vi "Set Channel Enable Mask.vi"(8 "error in (no error)":errorcluster, 10 "Channel Enable":bool[](array[boolean])=[FALSE, FALSE, FALSE, FALSE, FALSE, FALSE, FALSE, FALSE, FALSE, FALSE, FALSE, FALSE, FALSE, FALSE, FALSE, FALSE, FALSE, FALSE], 11 "LINX-SN3218 in":refnum<class "LINX-SN3218.lvclass">) -> (0 "error out":errorcluster, 3 "LINX-SN3218 out":refnum<class "LINX-SN3218.lvclass">)   [LabVIEW 2020, in "LINX-SN3218.lvclass"]
uses:
  LINX-SN3218.lvclass
  LINX I2C/LINX I2C.lvclass
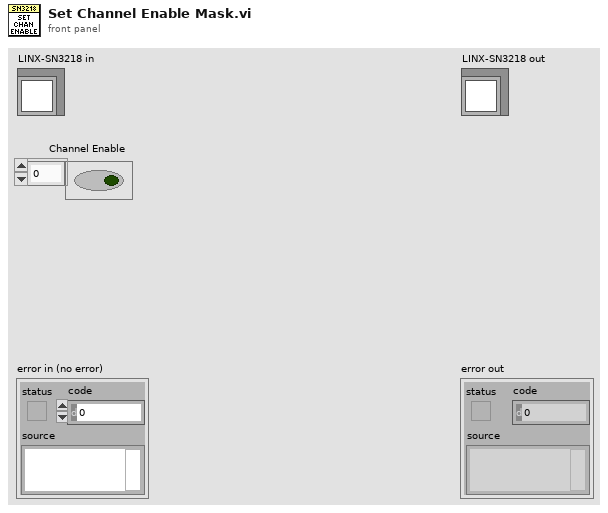
[diagram p1: front panel]
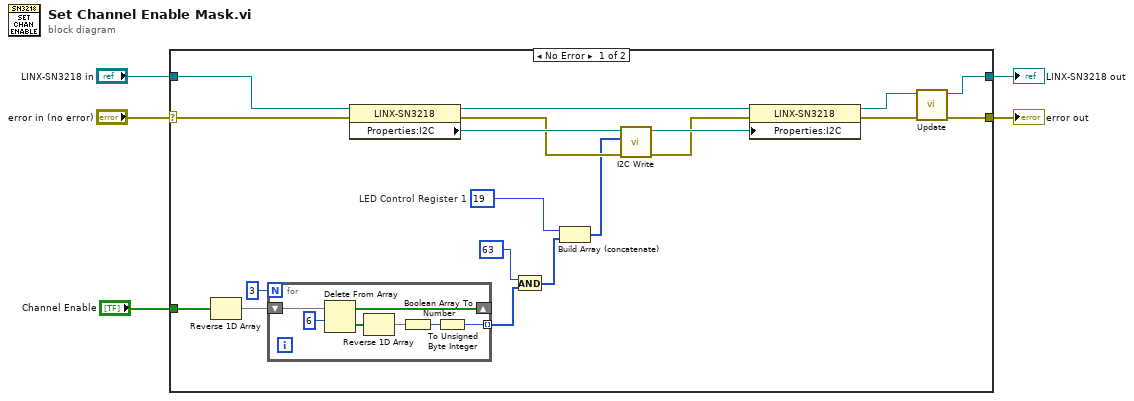
[diagram p0: block diagram]
diagram:
  n1 = case shown="No Error" "error in (no error)" {
    selector: "error in (no error)" -> [w22 w33]
    tunnel: [w11 w33] -> w4
    tunnel: [w10 w32] -> w2
    tunnel: "LINX-SN3218 in" -> [w24 w32]
    tunnel: "Channel Enable" -> [w9 _]
    frame No Error {
      w17 = u8 19  # LED Control Register 1
      n2 = Reverse 1D Array(array=w9) -> (reversed array=w6:bool[])
      n3 = for {
        N: 3 -> [_]
        shift-right: [w30] -> _
        shift-left: w6 -> [w31]
        tunnel: [w26] -> w7 mode=indexing
        n4 = Delete From Array(array=w31, length=6) -> (deleted portion=w28:bool[], array with subset deleted=w30:bool[])  [unwired: 1 in]
        n5 = Reverse 1D Array(array=w28) -> (reversed array=w25:bool[])
        n6 = Boolean Array To Number(Boolean array=w25) -> (number=w27:u32)
        n7 = To Unsigned Byte Integer(number=w27) -> (unsigned 8bit integer=w26:u8)
      }
      n8 = property class="LINX-SN3218"(reference=w24, error in=w22) -> (reference out=w21:refnum<class "LINX-SN3218.lvclass">, error out=w19:errorcluster, "Properties:I2C"=w23:refnum<class "LINX I2C.lvclass">)
      n9 = And(x=u8 63, y=w7) -> (x .and. y?=w14:u8[])
      n10 = Build Array (concatenate)(w17, w14) -> (w16:u8[])
      n11 = call "I2C Write.vi"("error in (no error)"=w19, "Bytes to Write"=w16, "LINX I2C in"=w23) -> ("error out"=w18:errorcluster, "LINX I2C out"=w20:refnum<class "LINX I2C.lvclass">)  [unwired: 7 in]
      n12 = property class="LINX-SN3218"(reference=w21, error in=w18, "Properties:I2C"=w20) -> (reference out=w12:refnum<class "LINX-SN3218.lvclass">, error out=w13:errorcluster)
      n13 = call "Update.vi"("error in (no error)"=w13, "LINX-SN3218 in"=w12) -> ("error out"=w11:errorcluster, "LINX-SN3218 out"=w10:refnum<class "LINX-SN3218.lvclass">)  [unwired: 8 in]
    }
    frame Error {
    }
  }
  "error out" <- w4
  "LINX-SN3218 out" <- w2
